vi "VAC_Measure.vi"() -> ()   [LabVIEW 2018]
doc: "Read one the value of one analog channel from a LINX device."
uses:
  <vilib>/MakerHub/LINX/Public/Peripherals/Digital/Digital Write 1 Chan.vi
  <vilib>/MakerHub/LINX/Public/Peripherals/Analog/Analog Read 1 Chan.vi
  <vilib>/MakerHub/LINX/Public/Peripherals/Digital/Digital Write N Chans.vi
  <vilib>/MakerHub/LINX/Public/Peripherals/Analog/Analog Read N Chans.vi
  <vilib>/MakerHub/LINX/Private/Local IO/LinxDigitalWrite.vi
  <vilib>/MakerHub/LINX/Public/Utilities/Check Channel.vi
  <vilib>/MakerHub/LINX/Private/Local IO/LinxAnalogRead.vi
  <vilib>/MakerHub/LINX/Public/Utilities/Open Serial.vi
  <vilib>/MakerHub/LINX/Private/Utilties/Generate Error.vi
  <vilib>/MakerHub/LINX/LMH-LINX.lvlib
  LW/LIRA_toolbox.lvlib
panel:
  in  "Напряжение":T1={"Измеряемая величина"="U", "единицы измерения"="В", "Ширина строки (в символах)"="16", "Количество знаков после запятой"="2"}
  in  "Сила тока":T1={"Измеряемая величина"="I", "единицы измерения"="A", "Ширина строки (в символах)"="16", "Количество знаков после запятой"="2"}
  in  "Количество стрингов":i32=1
  in  "Название файла":string="1"
  in  "Путь к файлу с указанием на случайный txt файл":path=path "I:/Снятие_ВАХ/log/20250902_16_09_1.txt"
  in  "Старт":bool
  out "Numeric Control":i32
  out "Waveform Graph 2":dbl[](graph)
  out "Waveform Graph":dbl[](graph)
  out "Voltage":dbl
  out "Current":dbl
  out "array of clusters":cluster{"Voltage":dbl, "Voltage":dbl}[](array[cluster])
  out "XY Graph":cluster{"X":dbl, "Y":dbl}[](graph)
  in  "milliseconds to wait":u32=100
  in  "Charge C":bool
  in  "Discharge C":bool
  in  "connect FP":u8=31
  in  "discharge C":u8=30
  in  "I":u8=1
  in  "U":u8
  out "Loop Rate (Hz)":u32
  in  "Stop Button":bool
  in  "Serial Port":refnum<visa-resource-name>="COM6"
  # "Путь должен указывать на случайный txt файл"
  # "Analog Value"
  # "LINX Device Settings"
  # "Analog Read Example (Serial Interface)\n\nThis example demonstrates how to read analog input values from a LINX device connected to the host computer via Serial / USB.\n\nInstructions\n1. Select the COM Port associated with the LINX Device.\n2. Select the Analog Channel to read.\n3. Click the Run Arrow."
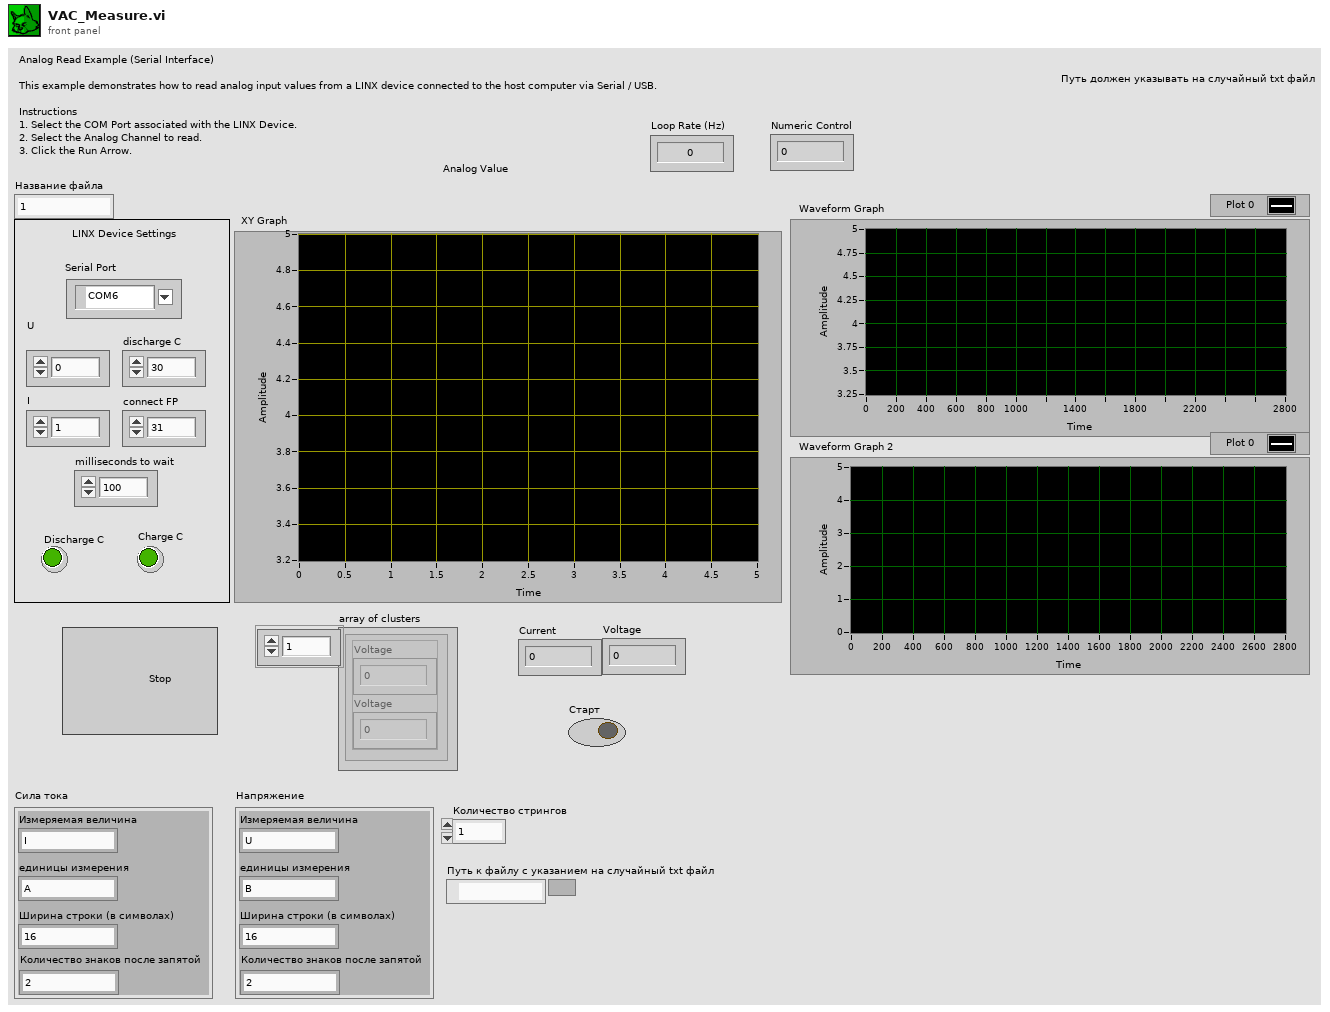
[diagram p1: front panel]
types:
  T1 = cluster{"Измеряемая величина":string, "единицы измерения":string, "Ширина строки (в символах)":string, "Количество знаков после запятой":string}
  T2 = typedef "LMH-LINX.lvlib/LINX Ref.ctl" = cluster{"IO":T3, "Interface":T4, "LINX Device Config":T5}
  T3 = typedef "LMH-LINX.lvlib/Platform.ctl" = enum16{"Remote", "Local"}
  T4 = typedef "LMH-LINX.lvlib/Interface.ctl" = enum16{"Serial", "TCP"}
  T5 = typedef "LMH-LINX.lvlib/Device.lvlib/LINX Device Config.ctl" = cluster{"Interface":T4, "COM Port":refnum<visa-resource-name>, "TCP Configuration":T6, "Device Family":u8, "Device ID":u8, "Device Name":string, "TCP Ref":refnum<k5>, "Channels":T7}
  T6 = typedef "LMH-LINX.lvlib/Device.lvlib/TCP Config.ctl" = cluster{"IP Address":string, "Port":u16}
  T7 = typedef "LMH-LINX.lvlib/Channels.ctl" = cluster{"DI":u8[], "DO":u8[], "AI":u8[], "AO":u8[], "PWM":u8[], "QE":u8[], "UART":u8[], "I2C 2":u8[], "SPI":u8[], "CAN":u8[], "Servo":u8[], "AI Ref (V)":dbl, "AI Resolution (Bits)":u8, "AO Ref (V)":dbl, "AO Resolution (Bits)":u8}
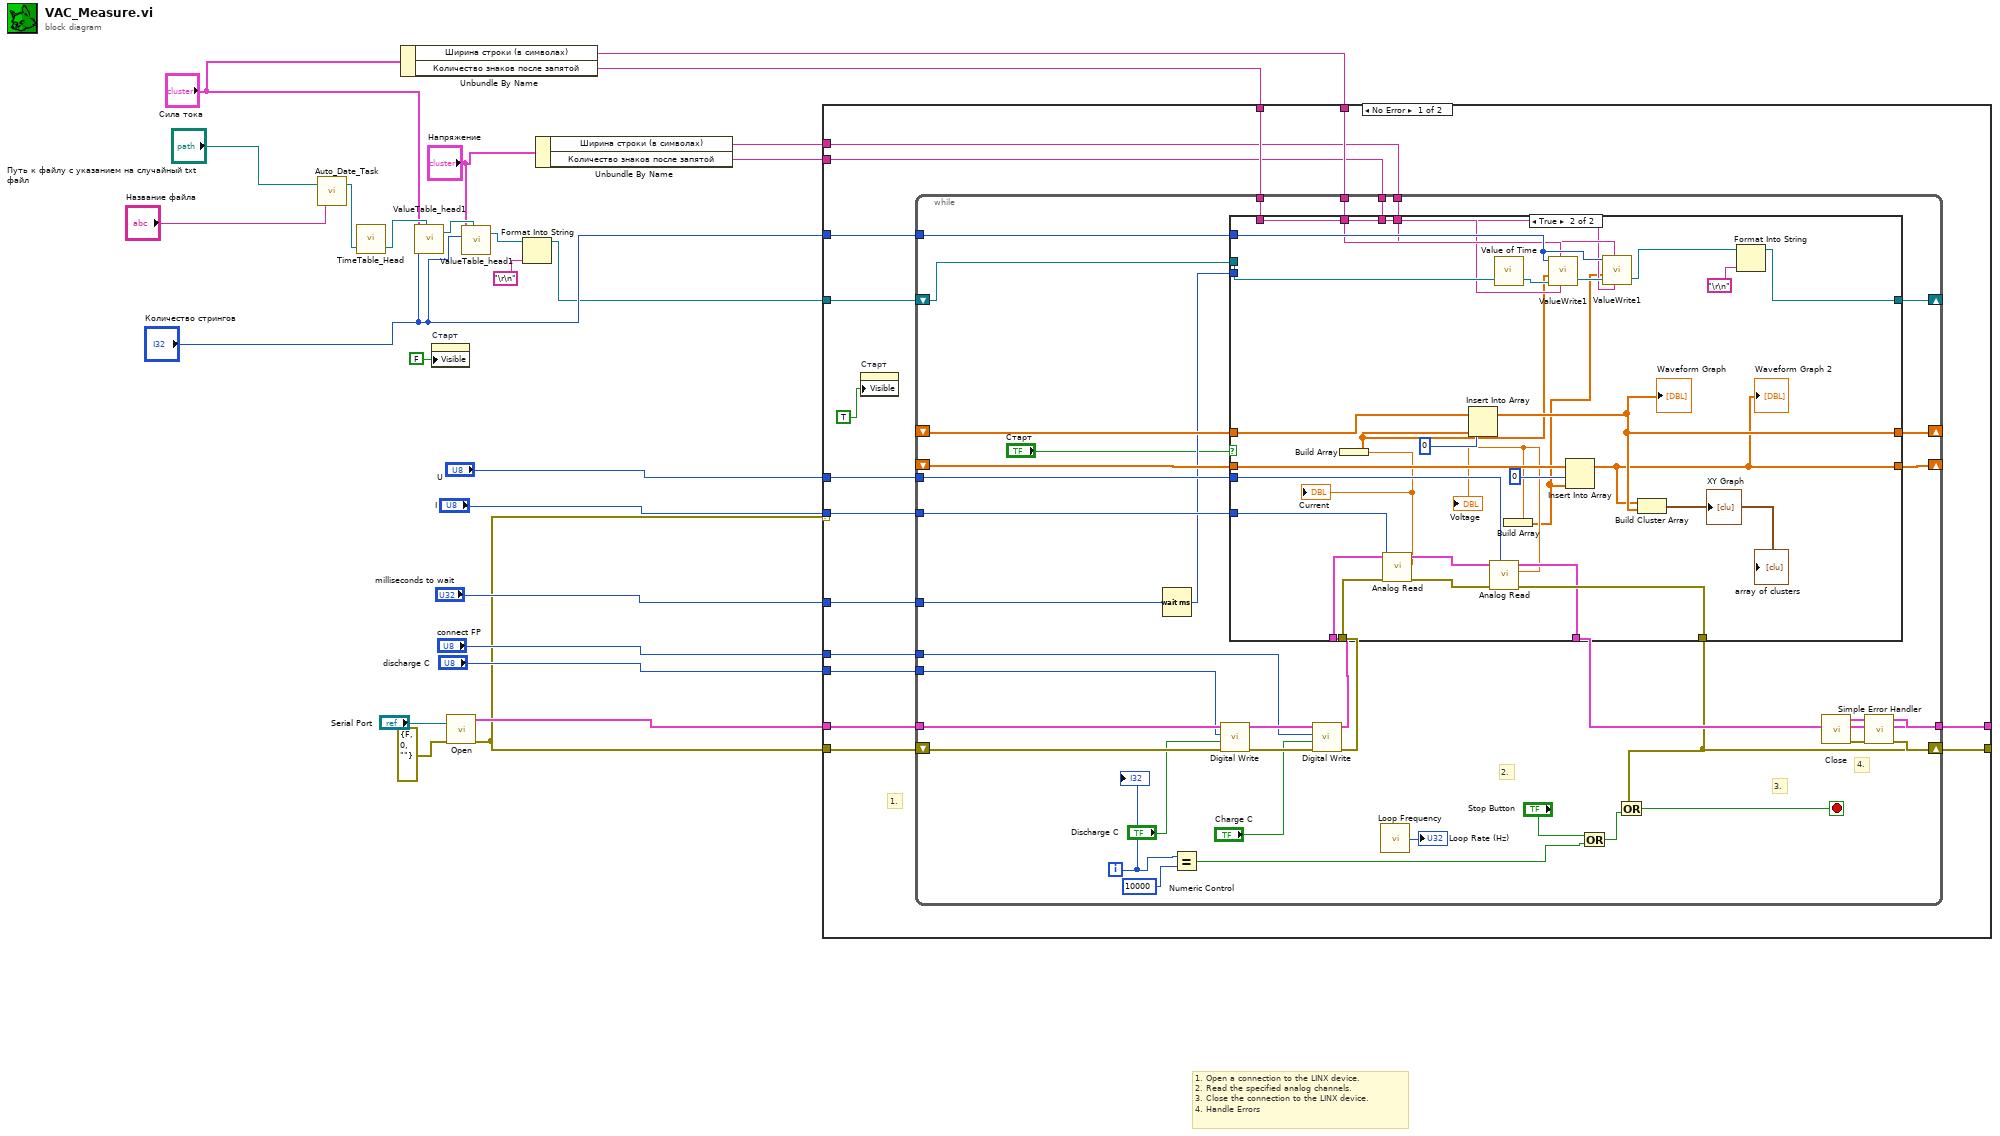
[diagram p0: block diagram]
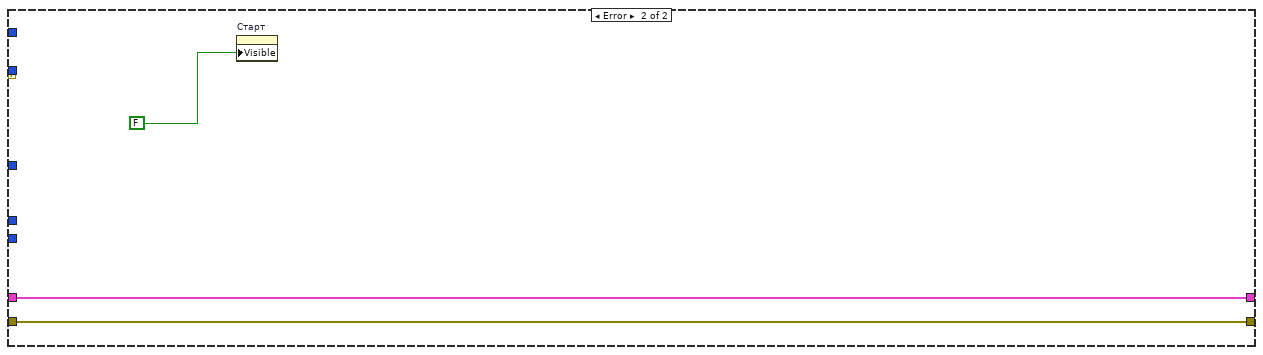
[diagram p3: hidden frame]
diagram:
  # "1. Open a connection to the LINX device.\n2. Read the specified analog channels.\n3. Close the connection to the LINX device.\n4. Handle Errors"
  # "4."
  n1 = call "Auto_Date_Task.vi"("Название файла"="Название файла", "Путь к файлу с указанием на случайный txt файл"="Путь к файлу с указанием на случайный txt файл") -> ("refnum out"=w13:refnum<file>)  [unwired: 1 out]
  n2 = call "TimeTable_Head.vi"("input file"=w13) -> ("output file refnum"=w12:refnum<file>)  [unwired: 1 in, 1 out]
  n3 = Unbundle By Name("Сила тока") -> ("Ширина строки (в символах)"=w8:string, "Количество знаков после запятой"=w7:string)
  n4 = call "ValueTable_head1.vi"("Файл записи"=w12, "Количество датчиков"="Количество стрингов", "Cluster"="Сила тока") -> ("Файл записи 2"=w11:refnum<file>)  [unwired: 3 in, 1 out]
  n5 = property on="Старт" class="Bool (strict)"("Visible"=FALSE) -> ()  [unwired: 2 in, 2 out]
  n6 = call-poly <vilib>:"Open.vi"("Error In"=errorcluster {"status"=FALSE, "code"=0, "source"=""}, "Serial Port"="Serial Port") -> ("Error Out"=w15:errorcluster, "LINX Resource"=w28:T2)  [unwired: 7 in, 1 out]
  n7 = call "ValueTable_head1.vi"("Файл записи"=w11, "Количество датчиков"="Количество стрингов", "Cluster"="Напряжение") -> ("Файл записи 2"=w2:refnum<file>)  [unwired: 3 in, 1 out]
  n8 = Format Into String(initial string=w2, "\r\n") -> (resulting string=w1:refnum<file>)  [unwired: 2 in, 1 out]
  n9 = Unbundle By Name("Напряжение") -> ("Ширина строки (в символах)"=w5:string, "Количество знаков после запятой"=w4:string)
  n10 = case shown="No Error" w15 {
    tunnel: w28 -> [w44 w116]
    tunnel: w15 -> [w43 w117]
    tunnel: [w42 w116] -> w27
    tunnel: "discharge C" -> [w41 _]
    tunnel: "connect FP" -> [w40 _]
    tunnel: "milliseconds to wait" -> [w39 _]
    tunnel: "I" -> [w38 _]
    tunnel: "U" -> [w37 _]
    tunnel: [w36 w117] -> w18
    tunnel: w1 -> [w35 _]
    tunnel: "Количество стрингов" -> [w33 _]
    tunnel: w8 -> [w32 _]
    tunnel: w7 -> [w31 _]
    tunnel: w5 -> [w30 _]
    tunnel: w4 -> [w29 _]
    frame No Error {
      # "3."
      # "1."
      n11 = property on="Старт" class="Bool (strict)"("Visible"=TRUE) -> ()  [unwired: 2 in, 2 out]
      n12 = while {
        tunnel: w44 -> [w78]
        tunnel: [w56] -> w42
        shift-right: [w55] -> w36
        shift-left: w43 -> [w76]
        tunnel: w41 -> [w74]
        tunnel: w40 -> [w73]
        tunnel: w39 -> [w72]
        shift-right: [w63] -> _
        shift-left: _ -> [w64]
        shift-right: [w62] -> _
        shift-left: _ -> [w65]
        tunnel: w38 -> [w59]
        tunnel: w37 -> [w57]
        shift-right: [w52] -> _
        shift-left: w35 -> [w50]
        tunnel: w33 -> [w49]
        tunnel: w32 -> [w48]
        tunnel: w31 -> [w47]
        tunnel: w30 -> [w46]
        tunnel: w29 -> [w45]
        i -> [w70]
        stop <- w54 stop-if-true
        # "2."
        n13 = Wait (ms)(milliseconds to wait=w72) -> (millisecond timer value=w53:u32)
        n14 = Equal?(x=w70, y=10000) -> (x = y?=w67:bool)
        n15 = call-poly <vilib>:"Digital Write.vi"("Error In"=w76, "Output Value"="Discharge C", "DO Channel"=w74, "LINX Resource"=w78) -> ("Error Out"=w75:errorcluster, "LINX Resource"=w77:T2)  [unwired: 6 in]
        n16 = call-poly <vilib>:"Digital Write.vi"("Error In"=w75, "Output Value"="Charge C", "DO Channel"=w73, "LINX Resource"=w77) -> ("Error Out"=w60:errorcluster, "LINX Resource"=w58:T2)  [unwired: 6 in]
        n17 = case shown="True" "Старт" {
          tunnel: w65 -> [w83 w112]
          tunnel: w64 -> [w84 w111]
          tunnel: [w84 w101] -> w63
          tunnel: [w83 w100] -> w62
          tunnel: w60 -> [w82 w110]
          tunnel: w59 -> [_ w109]
          tunnel: w58 -> [w81 w108]
          tunnel: w57 -> [_ w106]
          tunnel: [w82 w104] -> w55
          tunnel: [w81 w103] -> w56
          tunnel: w53 -> [_ _]
          tunnel: [w80 w85] -> w52
          tunnel: w50 -> [w80 w97]
          tunnel: w49 -> [_ w94]
          tunnel: w48 -> [_ w93]
          tunnel: w47 -> [_ w92]
          tunnel: w46 -> [_ w91]
          tunnel: w45 -> [_ w90]
          frame False {
          }
          frame True {
            n18 = call-poly <vilib>:"Analog Read.vi"("Error In"=w110, "Analog Channel"=w109, "LINX Resource"=w108) -> ("Error Out"=w107:errorcluster, "Voltage"=w99:dbl, "LINX Resource"=w105:T2)  [unwired: 5 in, 1 out]
            "Current" <- w99
            n19 = Build Array(w99) -> (w89:dbl[])
            n20 = Insert Into Array(array=w111, index=0, new element=w89) -> (w101:dbl[])
            "Waveform Graph" <- w101
            n21 = call-poly <vilib>:"Analog Read.vi"("Error In"=w107, "Analog Channel"=w106, "LINX Resource"=w105) -> ("Error Out"=w104:errorcluster, "Voltage"=w98:dbl, "LINX Resource"=w103:T2)  [unwired: 5 in, 1 out]
            "Voltage" <- w98
            n22 = call "Value of Time.vi"("input file"=w97) -> ("output file refnum"=w96:refnum<file>)  [unwired: 1 in, 1 out]
            n23 = Build Array(w98) -> (w88:dbl[])
            n24 = call "ValueWrite1.vi"("Количество знаков после запятой"=w92, "Ширина строки (в символах)"=w93, "Файл с заголовком"=w96, "Массив с измерениями"=w89, "Количество датчиков"=w94) -> ("Файл с заголовком 2"=w95:refnum<file>)  [unwired: 1 in, 1 out]
            n25 = Insert Into Array(array=w112, index=0, new element=w88) -> (w100:dbl[])
            "Waveform Graph 2" <- w100
            n26 = call "ValueWrite1.vi"("Количество знаков после запятой"=w90, "Ширина строки (в символах)"=w91, "Файл с заголовком"=w95, "Массив с измерениями"=w88, "Количество датчиков"=w94) -> ("Файл с заголовком 2"=w86:refnum<file>)  [unwired: 1 in, 1 out]
            n27 = Build Cluster Array(w100, w101) -> (→"XY Graph" →"array of clusters":cluster{"Voltage":dbl, "Voltage":dbl}[])
            n28 = Format Into String(initial string=w86, "\r\n") -> (resulting string=w85:refnum<file>)  [unwired: 2 in, 1 out]
          }
        }
        n29 = call <vilib>:"Loop Frequency.vi"() -> ("Loop Rate (Hz)"=→"Loop Rate (Hz)":u32)
        n30 = Or(x="Stop Button", y=w67) -> (x .or. y?=w66:bool)
        n31 = Or(x=w55, y=w66) -> (x .or. y?=w54:bool)
        "Numeric Control" <- w70
      }
    }
    frame Error {
      n32 = property on="Старт" class="Bool (strict)"("Visible"=FALSE) -> ()  [unwired: 2 in, 2 out]
    }
  }
  n33 = call <vilib>:"Close.vi"("Error In"=w18, "LINX Resource"=w27) -> ("Error Out"=w25:errorcluster)  [unwired: 9 in]
  n34 = call <vilib>:"Simple Error Handler.vi"("error in (no error)"=w25) -> ()  [unwired: 4 in, 5 out]
